vi "Determine Waveform Scan Name.vi"(8 "error in (no error)":errorcluster, 10 "Waveform Settings":T1, 11 "Model in":refnum<class "Model.lvclass">) -> (0 "error out":errorcluster, 2 "Waveform Scan Name":string, 3 "Model out":refnum<class "Model.lvclass">)   [LabVIEW 2015, in "Model.lvclass"]
uses:
  Model.lvclass
  Typedefs/Waveform Settings.ctl
  Typedefs/Waveform Types.ctl
  Typedefs/FAMT Typedefs.lvlib
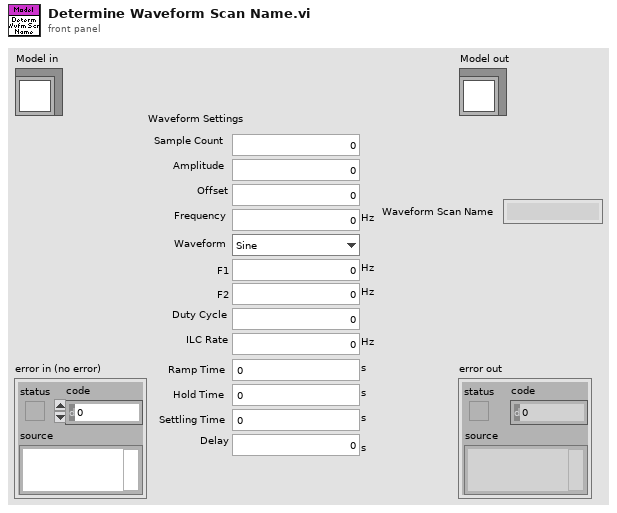
[diagram p1: front panel]
types:
  T1 = typedef "FAMT Typedefs.lvlib/Waveform Settings.ctl" = cluster{"Sample Count":u32, "Amplitude":dbl, "Offset":dbl, "Frequency":dbl[unit], "Waveform":T2, "F1":dbl[unit], "F2":dbl[unit], "Duty Cycle":dbl, "ILC Rate":dbl[unit], "Ramp Time":dbl[unit], "Hold Time":dbl[unit], "Settling Time":dbl[unit], "Delay":dbl[unit]}
  T2 = typedef "FAMT Typedefs.lvlib/Waveform Types.ctl" = enum16{"Sine", "Triangle", "Square", "Sawtooth", "Chirp", "Gaussian", "Trapezoid"}
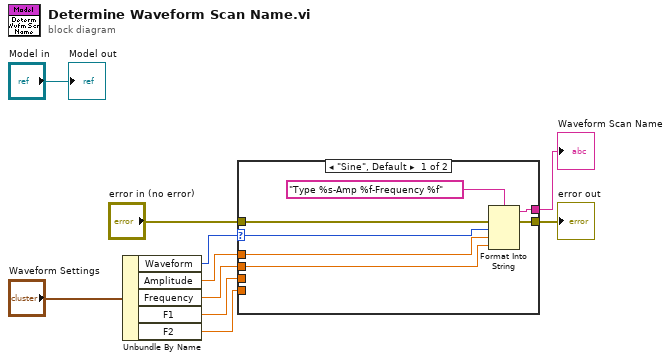
[diagram p0: block diagram]
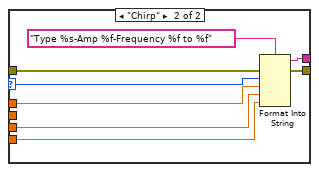
[diagram p2: hidden frame]
diagram:
  n1 = Unbundle By Name("Waveform Settings") -> ("Waveform"=w8:T2, "Amplitude"=w7:dbl, "Frequency"=w6:dbl[unit], "F1"=w5:dbl[unit], "F2"=w4:dbl[unit])
  n2 = case shown="\"Sine\", Default" w8 {
    selector: w8 -> [w14 w21]
    tunnel: w7 -> [w16 w22]
    tunnel: w6 -> [w15 _]
    tunnel: w5 -> [_ w24]
    tunnel: w4 -> [_ w23]
    tunnel: [w13 w20] -> w1
    tunnel: "error in (no error)" -> [w12 w19]
    tunnel: [w11 w18] -> w2
    frame "Sine", Default {
      n3 = Format Into String(format string="Type %s-Amp %f-Frequency %f", error in=w12, w14, w16, w15) -> (resulting string=w13:string, error out=w11:errorcluster)  [unwired: 1 in]
    }
    frame "Chirp" {
      n4 = Format Into String(format string="Type %s-Amp %f-Frequency %f to %f", error in=w19, w21, w22, w24, w23) -> (resulting string=w20:string, error out=w18:errorcluster)  [unwired: 1 in]
    }
  }
  "error out" <- w2
  "Waveform Scan Name" <- w1
  "Model out" <- "Model in"
